vi "Main.vi"() -> ()   [LabVIEW 2019]
uses:
  Controls/#enum_DeliveryType.ctl
  Factory/Factory.lvclass
  Controls/#cluster_PersonalData.ctl
panel:
  in  "Stop":bool
  in  "Order Shipping":bool
  in  "Delivery Type":T1
  in  "Weight [kg]":dbl
  in  "Recipient's Address":string
  in  "Sender's Address":string
  in  "Recipient's Name:":string
  in  "Sender's Name:":string
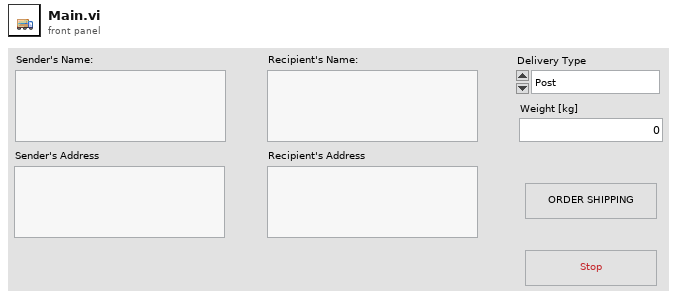
[diagram p1: front panel]
types:
  T1 = typedef "#enum_DeliveryType.ctl" = enum16{"Post", "Courier", "Pigeon"}
  T2 = typedef "#cluster_PersonalData.ctl" = cluster{"Name":string, "Address":string}
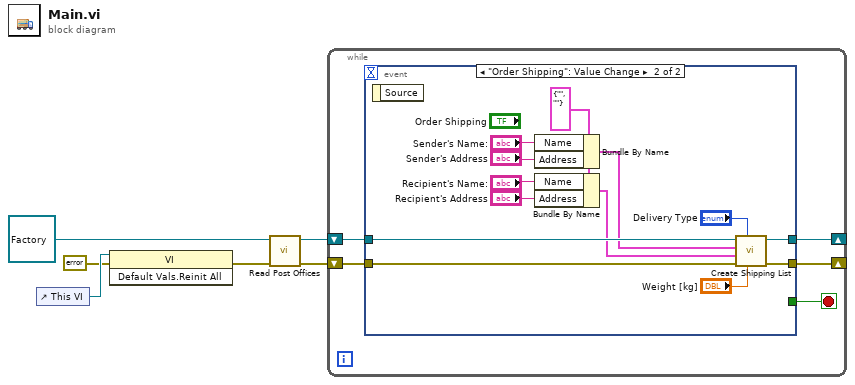
[diagram p0: block diagram]
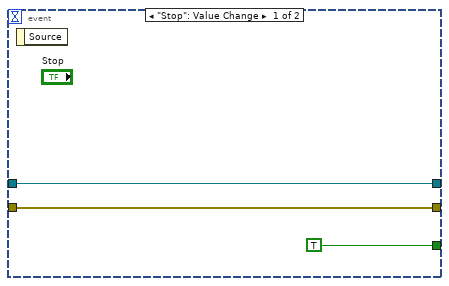
[diagram p2: hidden frame]
diagram:
  n1 = control-ref of="This VI"() -> (w6:refnum<vi>)
  n2 = invoke class="VI" method="Default Vals.Reinit All"(reference=w6, error in=errorcluster {"status"=FALSE, "code"=0, "source"=""} ("error out")) -> (error out=w4:errorcluster)  [unwired: 1 in, 2 out]
  n3 = call "Read Post Offices.vi"("error in (no error)"=w4, "Factory in"=refnum<class "Factory.lvclass"> refnum ("Factory.lvclass")) -> ("error out"=w2:errorcluster, "Factory out"=w1:refnum<class "Factory.lvclass">)  [unwired: 8 in]
  n4 = while {
    shift-right: [w7] -> _
    shift-left: w1 -> [w10]
    shift-right: [w9] -> _
    shift-left: w2 -> [w8]
    stop <- w11 stop-if-true
    n5 = event shown="[1] \"Order Shipping\": Value Change" {
      selector: _ -> [_ _]
      dyn-events: _ -> [_ _]
      timeout: _ -> [_ _]
      tunnel: [TRUE _] -> w11
      tunnel: w10 -> [w13 w27]
      tunnel: [w12 w19] -> w9
      tunnel: w8 -> [w12 w18]
      tunnel: [w13 w17] -> w7
      event "Stop": Value Change {
        n6 = event-data() -> ()  [unwired: 1 in, 1 out]
      }
      event "Order Shipping": Value Change {
        w24 = T2 {"Name"="", "Address"=""} ("Sender Data")
        n7 = event-data() -> ()  [unwired: 1 in, 1 out]
        n8 = Bundle By Name(cluster=w24, "Name"="Sender's Name:", "Address"="Sender's Address") -> (w21:T2)
        n9 = Bundle By Name(cluster=w24, "Name"="Recipient's Name:", "Address"="Recipient's Address") -> (w20:T2)
        n10 = call "Create Shipping List.vi"("Weight [kg]"="Weight [kg]", "Delivery Type"="Delivery Type", "error in (no error)"=w18, "Recipient Data"=w20, "Sender Data"=w21, "Factory in"=w27) -> ("error out"=w19:errorcluster, "Factory out"=w17:refnum<class "Factory.lvclass">)  [unwired: 4 in]
      }
    }
  }
